vi "Integrator Start-Stop.vi"(8 "error in (no error)":errorcluster, 9 "Start/Stop (F: Stop)":bool, 10 "Element (All: 0)":T1(ring), 11 "Yokogawa WT1600 in":refnum<class "Yokogawa WT1600.lvclass">) -> (0 "error out":errorcluster, 2 "VISA session":refnum<visa-resource-name>, 3 "Yokogawa WT1600 out":refnum<class "Yokogawa WT1600.lvclass">)   [LabVIEW 2013, in "Universal Power Meter.lvlib" / "Yokogawa WT1600.lvlib" / "Yokogawa WT1600.lvclass"]
uses:
  Yokogawa WT1600.lvclass
  Universal Power Meter class/Universal Power Meter.lvclass
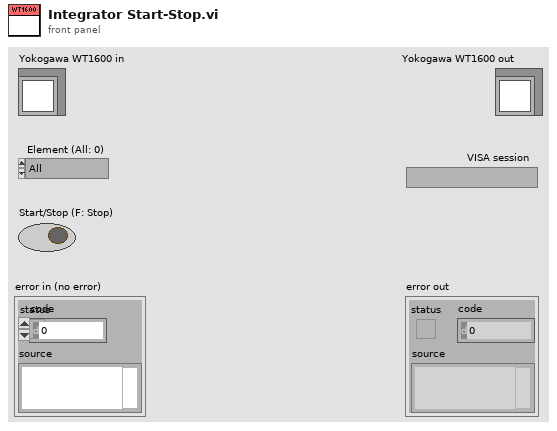
[diagram p1: front panel]
types:
  T1 = enum16{"All", "Element 1", "Element 2", "Element 3", "Element 4", "Element 5", "Element 6"}
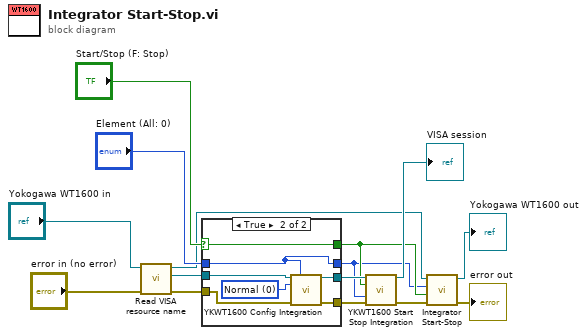
[diagram p0: block diagram]
diagram:
  n1 = call-dynamic "Read VISA resource name.vi"("error in (no error)"="error in (no error)", "Generic Instrument in"="Yokogawa WT1600 in") -> ("error out"=w6:errorcluster, "VISA resource name"=w8:refnum<visa-resource-name>, "Generic Instrument out"=w9:refnum<class "Yokogawa WT1600.lvclass">)  [unwired: 7 in]
  n2 = case shown="True" "Start/Stop (F: Stop)" {
    selector: "Start/Stop (F: Stop)" -> [w17 w21]
    tunnel: w8 -> [w19 w23]
    tunnel: w6 -> [w18 w25]
    tunnel: [w18 w24] -> w12
    tunnel: [w19 w22] -> w13
    tunnel: "Element (All: 0)" -> [w16 w20]
    tunnel: [w17 w21] -> w2
    tunnel: [w16 w20] -> w1
    frame False {
    }
    frame True {
      w26 = u16 0 items=["Normal", "Continuous"] ("Integ Mode (0: Normal)")
      n3 = call <instrlib>:"YKWT1600 Config Integration.vi"("VISA session"=w23, "Element (0: All)"=w20, "Integ Mode (0: Normal)"=w26, "error in (no error)"=w25) -> ("dup VISA session"=w22:refnum<visa-resource-name>, "error out"=w24:errorcluster)  [unwired: 10 in]
    }
  }
  n4 = call <instrlib>:"YKWT1600 Start Stop Integration.vi"("VISA session"=w13, "Start/Stop (F: Stop)"=w2, "Element (All: 0)"=w1, "error in (no error)"=w12) -> ("dup VISA session"=→"VISA session":refnum<visa-resource-name>, "error out"=w4:errorcluster)  [unwired: 10 in]
  n5 = call-parent "Integrator Start-Stop.vi"("error in (no error)"=w4, "Start/Stop (F: Stop)"=w2, "Element (All: 0)"=w1, "Universal Power Meter in"=w9) -> ("error out"=→"error out":errorcluster, "Universal Power Meter out"=→"Yokogawa WT1600 out":refnum<class "Yokogawa WT1600.lvclass">)  [unwired: 5 in, 1 out]
